vi "Timer2go.vi"() -> ()   [LabVIEW 2011]
uses:
  Control 1.ctl
panel:
  out "成功連結定時器":bool
  in  "stop 2":bool
  out "Today#2? \n(True=Enable)":bool
  out "now weekstring string":string
  out "after substring":string
  out "confilct ? (True=no conflict) 2":bool
  in  "Mon#2":bool
  in  "Tue#2":bool
  in  "Wed#2":bool
  in  "Thu#2":bool
  in  "Fri#2":bool
  in  "Sat#2":bool
  in  "Sun#2":bool
  in  "ON hour#2":i32
  in  "ON minute#2":i32
  in  "OFF hour#2":i32
  in  "OFF minute#2":i32
  out "week string#2":string
  out "ON hr+min#2":i32
  out "OFF hr+min#2":i32
  out "String":string
  out "path string":string
  out "read text":string
  out "CurrentPath":path=path "C:/Documents and Settings/TGI0362/My Documents/xUserData/LabVIEW_8.x/cmDVT_Factory-BBU-R5"
  in  "save":bool
  in  "error in":errorcluster
  in  "stop":bool
  out "error out 2":errorcluster
  out "VISA resource name out":refnum<visa-resource-name>
  out "error out":errorcluster
  out "VISA resource 2":refnum<visa-resource-name>
  out "定時器開啟":T1
  out "In Range?":bool
  out "hr+min":i32
  out "OFF hr+min#1":i32
  out "ON hr+min#1":i32
  out "Today#1? \n(True=Enable)":bool
  out "week string#1":string
  out "now week string":string
  out "confilct ? (True=no conflict)":bool
  in  "OFF minute#1":i32
  in  "OFF hour#1":i32
  in  "ON minute#1":i32
  in  "ON hour#1":i32
  in  "Sun#1":bool
  in  "Sat#1":bool
  in  "Fri#1":bool
  in  "Thu#1":bool
  in  "Wed#1":bool
  in  "Tue#1":bool
  in  "Mon#1":bool
  out "new picture":picture
  # "第一組\n\n\n第二組"
  # "："
  # "："
  # "："
  # "："
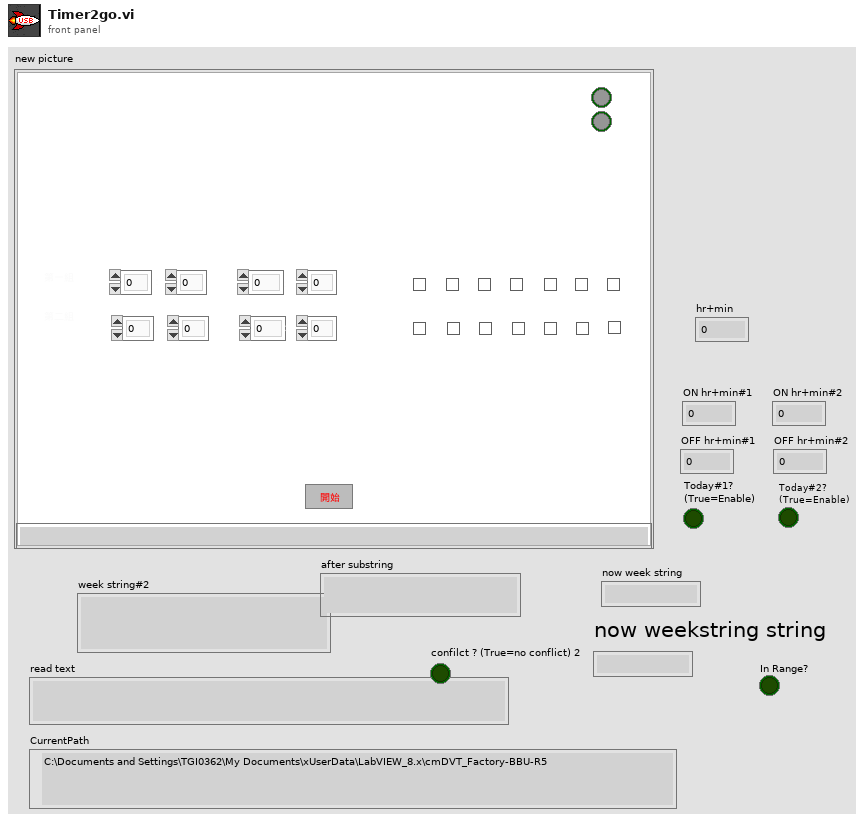
[diagram p1: front panel]
types:
  T1 = typedef "Control 1.ctl" = bool
  T2 = typedef "imagedata.ctl" = cluster{"image type":i32, "image depth":i32, "image":u8[], "mask":u8[], "colors":u32[], "Rectangle":cluster{"left":i16, "top":i16, "right":i16, "bottom":i16}}
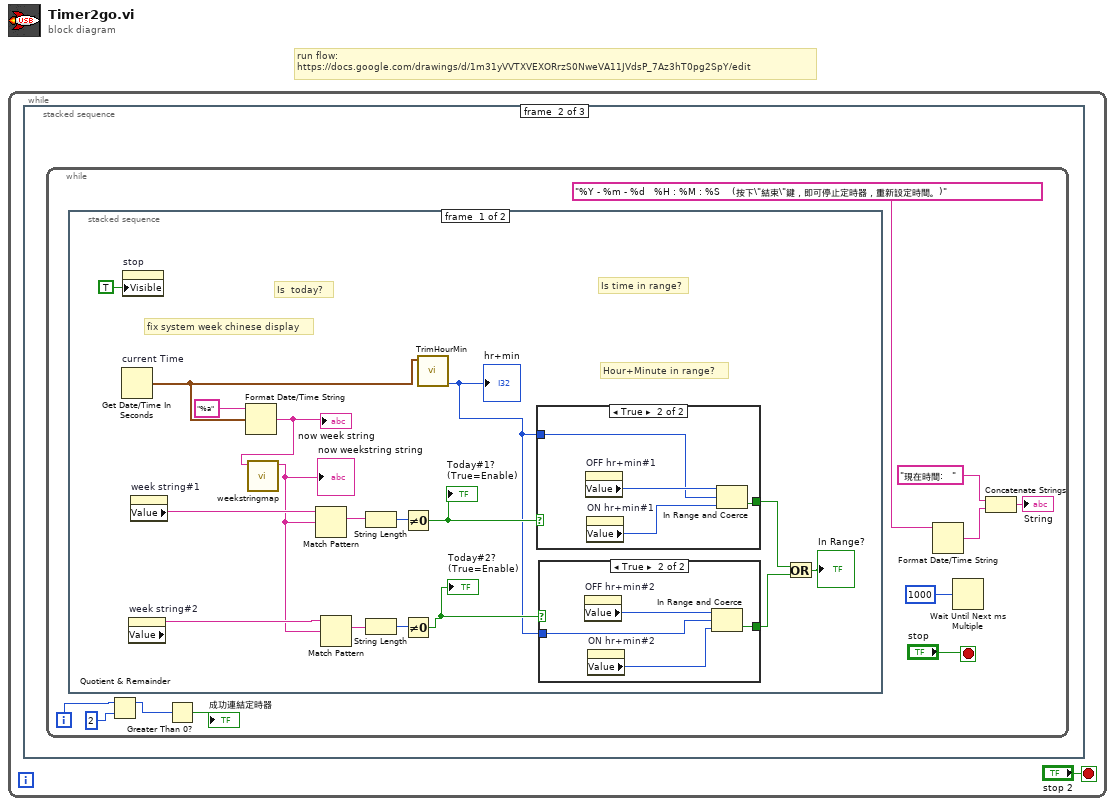
[diagram p0: block diagram]
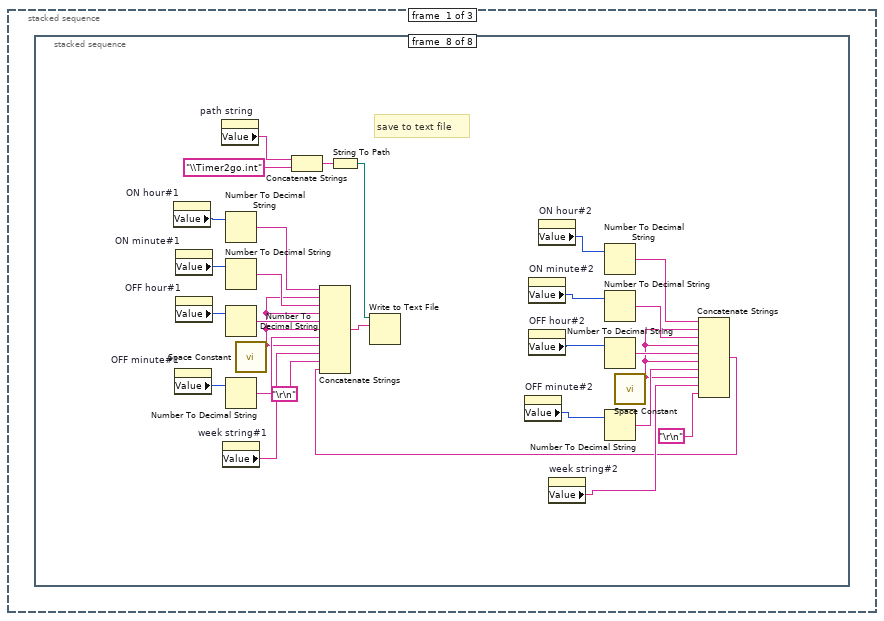
[diagram p2: hidden frame]
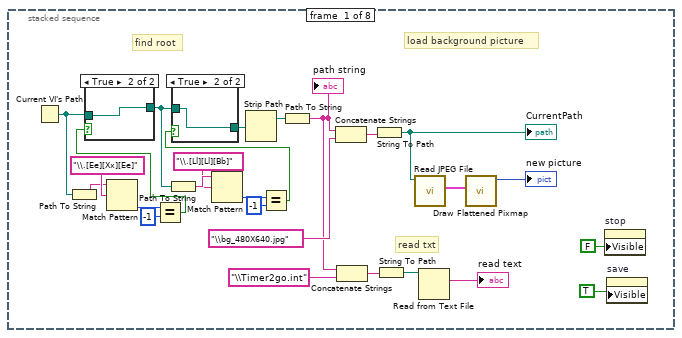
[diagram p3: hidden frame]
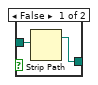
[diagram p4: hidden frame]
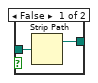
[diagram p5: hidden frame]
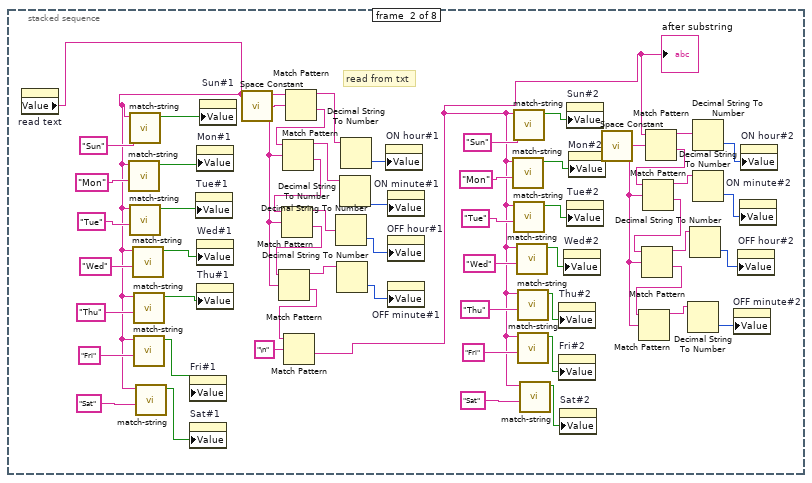
[diagram p6: hidden frame]
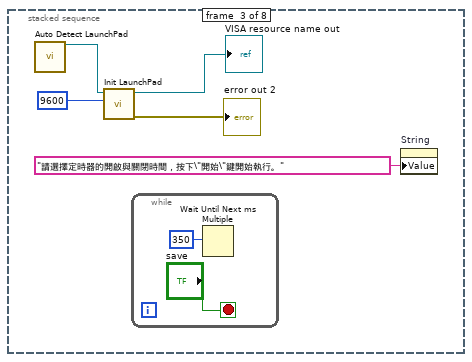
[diagram p7: hidden frame]
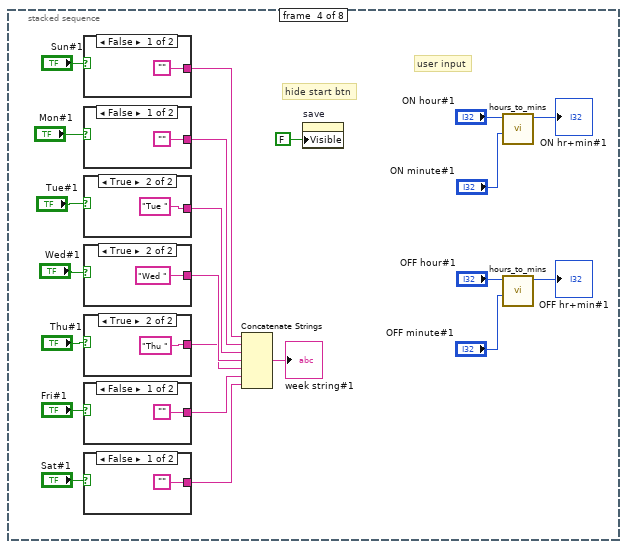
[diagram p8: hidden frame]
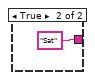
[diagram p9: hidden frame]
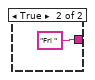
[diagram p10: hidden frame]
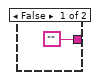
[diagram p11: hidden frame]
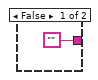
[diagram p12: hidden frame]
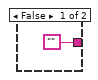
[diagram p13: hidden frame]
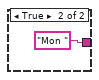
[diagram p14: hidden frame]
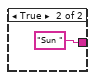
[diagram p15: hidden frame]
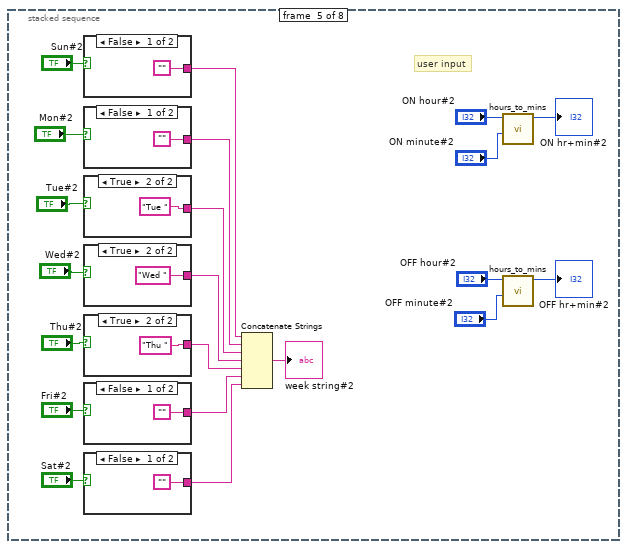
[diagram p16: hidden frame]
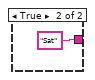
[diagram p17: hidden frame]
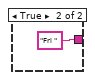
[diagram p18: hidden frame]
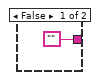
[diagram p19: hidden frame]
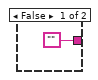
[diagram p20: hidden frame]
diagram:
  # "run flow:\nhttps://docs.google.com/drawings/d/1m31yVVTXVEXORrzS0NweVA11JVdsP_7Az3hT0pg2SpY/edit"
  n1 = while {
    stop <- "stop 2" stop-if-true
    n2 = stacked-sequence {
      frame #0 {
        n3 = stacked-sequence {
          frame #0 {
            # "read txt"
            # "load background picture"
            # "find root"
            n4 = Current VI's Path() -> (path=w16:path)
            n5 = Path To String(path=w16) -> (string=w15:string)
            n6 = Match Pattern(string=w15, regular expression="\\.[Ee][Xx][Ee]") -> (offset past match=w13:i32)  [unwired: 1 in, 3 out]
            n7 = Equal?(x=w13, y=-1) -> (x = y?=w25:bool)
            n8 = case shown="True" w25 {
              tunnel: [w31 w33] -> w22
              tunnel: w16 -> [w32 w33]
              frame False {
                n9 = Strip Path(path=w32) -> (stripped path=w31:path)  [unwired: 1 out]
              }
              frame True {
              }
            }
            n10 = Path To String(path=w22) -> (string=w19:string)
            n11 = Match Pattern(string=w19, regular expression="\\.[Ll][Ll][Bb]") -> (offset past match=w21:i32)  [unwired: 1 in, 3 out]
            n12 = Equal?(x=w21, y=-1) -> (x = y?=w24:bool)
            n13 = case shown="True" w24 {
              tunnel: [w28 w30] -> w23
              tunnel: w22 -> [w29 w30]
              frame False {
                n14 = Strip Path(path=w29) -> (stripped path=w28:path)  [unwired: 1 out]
              }
              frame True {
              }
            }
            n15 = Strip Path(path=w23) -> (stripped path=w12:path)  [unwired: 1 out]
            n16 = Path To String(path=w12) -> (string=w2:string)
            "path string" <- w2
            n17 = Concatenate Strings(w2, "\\bg_480X640.jpg") -> (w10:string)
            n18 = Concatenate Strings(w2, "\\Timer2go.int") -> (w5:string)
            n19 = String To Path(string=w10) -> (path=w9:path)
            "CurrentPath" <- w9
            n20 = String To Path(string=w5) -> (path=w4:path)
            n21 = call <vilib>:"Read JPEG File.vi"("path to JPEG file"=w9) -> ("image data"=w26:T2)  [unwired: 8 in, 2 out]
            n22 = Read from Text File(file (use dialog)=w4) -> (text=→"read text":string)  [unwired: 3 in, 3 out]
            n23 = call <vilib>:"Draw Flattened Pixmap.vi"("image data"=w26) -> ("new picture"=→"new picture":picture)  [unwired: 8 in]
            n24 = property on="stop" class="Bool"("Visible"=FALSE) -> ()  [unwired: 2 in, 2 out]
            n25 = property on="save" class="Bool"("Visible"=TRUE) -> ()  [unwired: 2 in, 2 out]
          }
          frame #1 {
            # "read from txt"
            n26 = property on="read text" class="Str"() -> ("Value"=w37:string)  [unwired: 2 in, 2 out]
            n27 = call "match-string.vi"("match string"="Mon", "String"=w37) -> ("match?(True=match)"=w76:bool)  [unwired: 9 in]
            n28 = call "match-string.vi"("match string"="Sun", "String"=w37) -> ("match?(True=match)"=w89:bool)  [unwired: 9 in]
            n29 = call "match-string.vi"("match string"="Tue", "String"=w37) -> ("match?(True=match)"=w77:bool)  [unwired: 9 in]
            n30 = call "match-string.vi"("match string"="Wed", "String"=w37) -> ("match?(True=match)"=w78:bool)  [unwired: 9 in]
            n31 = call "match-string.vi"("match string"="Thu", "String"=w37) -> ("match?(True=match)"=w79:bool)  [unwired: 9 in]
            n32 = call "match-string.vi"("match string"="Fri", "String"=w37) -> ("match?(True=match)"=w80:bool)  [unwired: 9 in]
            n33 = call "match-string.vi"("match string"="Sat", "String"=w37) -> ("match?(True=match)"=w81:bool)  [unwired: 9 in]
            n34 = property on="Fri#1" class="Bool (strict)"("Value"=w80) -> ()  [unwired: 2 in, 2 out]
            n35 = property on="Sat#1" class="Bool (strict)"("Value"=w81) -> ()  [unwired: 2 in, 2 out]
            n36 = property on="Tue#1" class="Bool (strict)"("Value"=w77) -> ()  [unwired: 2 in, 2 out]
            n37 = property on="Mon#1" class="Bool (strict)"("Value"=w76) -> ()  [unwired: 2 in, 2 out]
            n38 = property on="Wed#1" class="Bool (strict)"("Value"=w78) -> ()  [unwired: 2 in, 2 out]
            n39 = property on="Thu#1" class="Bool (strict)"("Value"=w79) -> ()  [unwired: 2 in, 2 out]
            n40 = property on="Sun#1" class="Bool (strict)"("Value"=w89) -> ()  [unwired: 2 in, 2 out]
            n41 = call <vilib>:"Space Constant.vi"() -> ("String"=w65:string)
            n42 = Match Pattern(string=w37, regular expression=w65) -> (before substring=w75:string, after substring=w73:string)  [unwired: 1 in, 2 out]
            n43 = Match Pattern(string=w73, regular expression=w65) -> (before substring=w72:string, after substring=w71:string)  [unwired: 1 in, 2 out]
            n44 = Match Pattern(string=w71, regular expression=w65) -> (before substring=w70:string, after substring=w67:string)  [unwired: 1 in, 2 out]
            n45 = Match Pattern(string=w67, regular expression=w65) -> (before substring=w66:string, after substring=w36:string)  [unwired: 1 in, 2 out]
            n46 = Match Pattern(string=w36, regular expression="\n") -> (after substring=w34:string)  [unwired: 1 in, 3 out]
            "after substring" <- w34
            n47 = Decimal String To Number(string=w70) -> (number=w69:i32)  [unwired: 2 in, 1 out]
            n48 = Decimal String To Number(string=w66) -> (number=w64:i32)  [unwired: 2 in, 1 out]
            n49 = Decimal String To Number(string=w72) -> (number=w68:i32)  [unwired: 2 in, 1 out]
            n50 = Decimal String To Number(string=w75) -> (number=w74:i32)  [unwired: 2 in, 1 out]
            n51 = property on="ON hour#1" class="DigNum (strict)"("Value"=w74) -> ()  [unwired: 2 in, 2 out]
            n52 = property on="ON minute#1" class="DigNum (strict)"("Value"=w68) -> ()  [unwired: 2 in, 2 out]
            n53 = property on="OFF hour#1" class="DigNum (strict)"("Value"=w69) -> ()  [unwired: 2 in, 2 out]
            n54 = property on="OFF minute#1" class="DigNum (strict)"("Value"=w64) -> ()  [unwired: 2 in, 2 out]
            n55 = call "match-string.vi"("match string"="Mon", "String"=w34) -> ("match?(True=match)"=w55:bool)  [unwired: 9 in]
            n56 = call "match-string.vi"("match string"="Sun", "String"=w34) -> ("match?(True=match)"=w56:bool)  [unwired: 9 in]
            n57 = call "match-string.vi"("match string"="Tue", "String"=w34) -> ("match?(True=match)"=w54:bool)  [unwired: 9 in]
            n58 = call "match-string.vi"("match string"="Wed", "String"=w34) -> ("match?(True=match)"=w53:bool)  [unwired: 9 in]
            n59 = call "match-string.vi"("match string"="Thu", "String"=w34) -> ("match?(True=match)"=w52:bool)  [unwired: 9 in]
            n60 = call "match-string.vi"("match string"="Fri", "String"=w34) -> ("match?(True=match)"=w51:bool)  [unwired: 9 in]
            n61 = call "match-string.vi"("match string"="Sat", "String"=w34) -> ("match?(True=match)"=w50:bool)  [unwired: 9 in]
            n62 = property on="Thu#2" class="Bool (strict)"("Value"=w52) -> ()  [unwired: 2 in, 2 out]
            n63 = property on="Fri#2" class="Bool (strict)"("Value"=w51) -> ()  [unwired: 2 in, 2 out]
            n64 = property on="Sat#2" class="Bool (strict)"("Value"=w50) -> ()  [unwired: 2 in, 2 out]
            n65 = property on="Wed#2" class="Bool (strict)"("Value"=w53) -> ()  [unwired: 2 in, 2 out]
            n66 = property on="Sun#2" class="Bool (strict)"("Value"=w56) -> ()  [unwired: 2 in, 2 out]
            n67 = property on="Tue#2" class="Bool (strict)"("Value"=w54) -> ()  [unwired: 2 in, 2 out]
            n68 = property on="Mon#2" class="Bool (strict)"("Value"=w55) -> ()  [unwired: 2 in, 2 out]
            n69 = call <vilib>:"Space Constant.vi"() -> ("String"=w38:string)
            n70 = Match Pattern(string=w34, regular expression=w38) -> (before substring=w49:string, after substring=w48:string)  [unwired: 1 in, 2 out]
            n71 = Match Pattern(string=w48, regular expression=w38) -> (before substring=w47:string, after substring=w46:string)  [unwired: 1 in, 2 out]
            n72 = Match Pattern(string=w46, regular expression=w38) -> (before substring=w45:string, after substring=w44:string)  [unwired: 1 in, 2 out]
            n73 = Match Pattern(string=w44, regular expression=w38) -> (before substring=w43:string)  [unwired: 1 in, 3 out]
            n74 = Decimal String To Number(string=w43) -> (number=w39:i32)  [unwired: 2 in, 1 out]
            n75 = Decimal String To Number(string=w45) -> (number=w40:i32)  [unwired: 2 in, 1 out]
            n76 = Decimal String To Number(string=w49) -> (number=w42:i32)  [unwired: 2 in, 1 out]
            n77 = Decimal String To Number(string=w47) -> (number=w41:i32)  [unwired: 2 in, 1 out]
            n78 = property on="OFF minute#2" class="DigNum (strict)"("Value"=w39) -> ()  [unwired: 2 in, 2 out]
            n79 = property on="OFF hour#2" class="DigNum (strict)"("Value"=w40) -> ()  [unwired: 2 in, 2 out]
            n80 = property on="ON minute#2" class="DigNum (strict)"("Value"=w41) -> ()  [unwired: 2 in, 2 out]
            n81 = property on="ON hour#2" class="DigNum (strict)"("Value"=w42) -> ()  [unwired: 2 in, 2 out]
          }
          frame #2 {
            n82 = call "Auto Detect LaunchPad.vi"() -> ("VISA resource"=w93:refnum<visa-resource-name>)  [unwired: 14 in, 1 out]
            n83 = call "Init LaunchPad.vi"("Baud Rate (9600)"=u32 9600, "VISA resource"=w93) -> ("error out"=→"error out 2":errorcluster, "VISA resource name out"=→"VISA resource name out":refnum<visa-resource-name>)  [unwired: 8 in]
            n84 = while {
              stop <- "save" stop-if-true
              n85 = Wait Until Next ms Multiple(millisecond multiple=u32 350) -> ()  [unwired: 1 out]
            }
            n86 = property on="String" class="Str"("Value"="請選擇定時器的開啟與關閉時間，按下\"開始\"鍵開始執行。" ("String")) -> ()  [unwired: 2 in, 2 out]
          }
          frame #3 {
            # "hide start btn"
            # "user input"
            n87 = case shown="False" "Sun#1" {
              tunnel: ["" "Sun "] -> w117
              frame False {
              }
              frame True {
              }
            }
            n88 = case shown="False" "Mon#1" {
              tunnel: ["" "Mon "] -> w110
              frame False {
              }
              frame True {
              }
            }
            n89 = case shown="True" "Tue#1" {
              tunnel: ["" "Tue "] -> w109
              frame False {
              }
              frame True {
              }
            }
            n90 = case shown="True" "Wed#1" {
              tunnel: ["" "Wed "] -> w108
              frame False {
              }
              frame True {
              }
            }
            n91 = case shown="True" "Thu#1" {
              tunnel: ["" "Thu "] -> w107
              frame False {
              }
              frame True {
              }
            }
            n92 = case shown="False" "Fri#1" {
              tunnel: ["" "Fri "] -> w106
              frame False {
              }
              frame True {
              }
            }
            n93 = case shown="False" "Sat#1" {
              tunnel: ["" "Sat"] -> w105
              frame False {
              }
              frame True {
              }
            }
            n94 = Concatenate Strings(w117, w110, w109, w108, w107, w106, w105) -> (→"week string#1":string)
            n95 = property on="save" class="Bool"("Visible"=FALSE) -> ()  [unwired: 2 in, 2 out]
            n96 = call "hours_to_mins.vi"("minute(00-59)"="ON minute#1", "hour(00-23)"="ON hour#1") -> ("hr+min"=→"ON hr+min#1":i32)  [unwired: 9 in]
            n97 = call "hours_to_mins.vi"("minute(00-59)"="OFF minute#1", "hour(00-23)"="OFF hour#1") -> ("hr+min"=→"OFF hr+min#1":i32)  [unwired: 9 in]
          }
          frame #4 {
            # "user input"
            n98 = case shown="False" "Sun#2" {
              tunnel: ["" "Sun "] -> w152
              frame False {
              }
              frame True {
              }
            }
            n99 = case shown="False" "Mon#2" {
              tunnel: ["" "Mon "] -> w145
              frame False {
              }
              frame True {
              }
            }
            n100 = case shown="True" "Tue#2" {
              tunnel: ["" "Tue "] -> w144
              frame False {
              }
              frame True {
              }
            }
            n101 = case shown="True" "Wed#2" {
              tunnel: ["" "Wed "] -> w143
              frame False {
              }
              frame True {
              }
            }
            n102 = case shown="True" "Thu#2" {
              tunnel: ["" "Thu "] -> w142
              frame False {
              }
              frame True {
              }
            }
            n103 = case shown="False" "Fri#2" {
              tunnel: ["" "Fri "] -> w141
              frame False {
              }
              frame True {
              }
            }
            n104 = case shown="False" "Sat#2" {
              tunnel: ["" "Sat"] -> w140
              frame False {
              }
              frame True {
              }
            }
            n105 = Concatenate Strings(w152, w145, w144, w143, w142, w141, w140) -> (→"week string#2":string)
            n106 = call "hours_to_mins.vi"("minute(00-59)"="ON minute#2", "hour(00-23)"="ON hour#2") -> ("hr+min"=→"ON hr+min#2":i32)  [unwired: 9 in]
            n107 = call "hours_to_mins.vi"("minute(00-59)"="OFF minute#2", "hour(00-23)"="OFF hour#2") -> ("hr+min"=→"OFF hr+min#2":i32)  [unwired: 9 in]
          }
          frame #5 {
            # "check Set Time conflict"
            n108 = property on="ON hour#1" class="DigNum (strict)"() -> ("Value"=w187:i32)  [unwired: 2 in, 2 out]
            n109 = property on="OFF hour#1" class="DigNum (strict)"() -> ("Value"=w190:i32)  [unwired: 2 in, 2 out]
            n110 = property on="ON minute#1" class="DigNum (strict)"() -> ("Value"=w184:i32)  [unwired: 2 in, 2 out]
            n111 = property on="OFF minute#1" class="DigNum (strict)"() -> ("Value"=w181:i32)  [unwired: 2 in, 2 out]
            n112 = Equal?(x=w190, y=0) -> (x = y?=w192:bool)
            n113 = Equal?(x=w187, y=0) -> (x = y?=w189:bool)
            n114 = case shown="False" w192 {
              tunnel: [w203 24] -> w177
              tunnel: w190 -> [w203 _]
              frame False {
              }
              frame True {
              }
            }
            n115 = case shown="False" w189 {
              tunnel: [w201 24] -> w171
              tunnel: w187 -> [w201 _]
              frame False {
              }
              frame True {
              }
            }
            n116 = Equal?(x=w181, y=0) -> (x = y?=w183:bool)
            n117 = Equal?(x=w184, y=0) -> (x = y?=w186:bool)
            n118 = case shown="False" w183 {
              tunnel: [w197 60] -> w174
              tunnel: w181 -> [w197 _]
              frame False {
              }
              frame True {
              }
            }
            n119 = case shown="False" w186 {
              tunnel: [w199 60] -> w169
              tunnel: w184 -> [w199 _]
              frame False {
              }
              frame True {
              }
            }
            n120 = Multiply(x=w177, y=60) -> (x*y=w175:i32)
            n121 = Multiply(x=w171, y=60) -> (x*y=w170:i32)
            n122 = Add(x=w175, y=w174) -> (x+y=w173:i32)
            n123 = Add(x=w170, y=w169) -> (x+y=w168:i32)
            n124 = Subtract(x=w177, y=w171) -> (x-y=w194:i32)
            n125 = Subtract(x=w173, y=w168) -> (x-y=w193:i32)
            n126 = Greater Or Equal To 0?(x=w194) -> (x >= 0?=w180:bool)
            n127 = Greater Than 0?(x=w193) -> (x > 0?=w179:bool)
            n128 = And(x=w180, y=w179) -> (x .and. y?=w178:bool)
            "confilct ? (True=no conflict)" <- w178
            n129 = case shown="True" w178 {
              frame False {
                n130 = One Button Dialog(message="time confilct!!") -> (true=w195:bool)  [unwired: 1 in]
                n131 = Stop(stop? (T)=w195) -> ()
              }
              frame True {
              }
            }
          }
          frame #6 {
            # "check Set Time conflict"
            n132 = property on="OFF minute#2" class="DigNum (strict)"() -> ("Value"=w207:i32)  [unwired: 2 in, 2 out]
            n133 = property on="ON hour#2" class="DigNum (strict)"() -> ("Value"=w206:i32)  [unwired: 2 in, 2 out]
            n134 = property on="OFF hour#2" class="DigNum (strict)"() -> ("Value"=w208:i32)  [unwired: 2 in, 2 out]
            n135 = property on="ON minute#2" class="DigNum (strict)"() -> ("Value"=w205:i32)  [unwired: 2 in, 2 out]
            n136 = Equal?(x=w208, y=0) -> (x = y?=w229:bool)
            n137 = Equal?(x=w206, y=0) -> (x = y?=w227:bool)
            n138 = case shown="False" w229 {
              tunnel: [w240 24] -> w218
              tunnel: w208 -> [w240 _]
              frame False {
              }
              frame True {
              }
            }
            n139 = case shown="False" w227 {
              tunnel: [w238 24] -> w212
              tunnel: w206 -> [w238 _]
              frame False {
              }
              frame True {
              }
            }
            n140 = Equal?(x=w207, y=0) -> (x = y?=w223:bool)
            n141 = Equal?(x=w205, y=0) -> (x = y?=w225:bool)
            n142 = case shown="False" w223 {
              tunnel: [w234 60] -> w215
              tunnel: w207 -> [w234 _]
              frame False {
              }
              frame True {
              }
            }
            n143 = case shown="False" w225 {
              tunnel: [w236 60] -> w210
              tunnel: w205 -> [w236 _]
              frame False {
              }
              frame True {
              }
            }
            n144 = Multiply(x=w218, y=60) -> (x*y=w216:i32)
            n145 = Multiply(x=w212, y=60) -> (x*y=w211:i32)
            n146 = Add(x=w216, y=w215) -> (x+y=w214:i32)
            n147 = Add(x=w211, y=w210) -> (x+y=w209:i32)
            n148 = Subtract(x=w218, y=w212) -> (x-y=w231:i32)
            n149 = Subtract(x=w214, y=w209) -> (x-y=w230:i32)
            n150 = Greater Or Equal To 0?(x=w231) -> (x >= 0?=w221:bool)
            n151 = Greater Than 0?(x=w230) -> (x > 0?=w220:bool)
            n152 = And(x=w221, y=w220) -> (x .and. y?=w219:bool)
            "confilct ? (True=no conflict) 2" <- w219
            n153 = case shown="True" w219 {
              frame False {
                n154 = One Button Dialog(message="time confilct!!") -> (true=w232:bool)  [unwired: 1 in]
                n155 = Stop(stop? (T)=w232) -> ()
              }
              frame True {
              }
            }
          }
          frame #7 {
            # "save to text file"
            n156 = property on="ON hour#1" class="DigNum (strict)"() -> ("Value"=w258:i32)  [unwired: 2 in, 2 out]
            n157 = property on="OFF minute#1" class="DigNum (strict)"() -> ("Value"=w255:i32)  [unwired: 2 in, 2 out]
            n158 = property on="ON minute#1" class="DigNum (strict)"() -> ("Value"=w257:i32)  [unwired: 2 in, 2 out]
            n159 = property on="OFF hour#1" class="DigNum (strict)"() -> ("Value"=w256:i32)  [unwired: 2 in, 2 out]
            n160 = property on="path string" class="Str"() -> ("Value"=w260:string)  [unwired: 2 in, 2 out]
            n161 = property on="week string#1" class="Str"() -> ("Value"=w265:string)  [unwired: 2 in, 2 out]
            n162 = Number To Decimal String(number=w258) -> (decimal integer string=w269:string)  [unwired: 1 in]
            n163 = Number To Decimal String(number=w257) -> (decimal integer string=w268:string)  [unwired: 1 in]
            n164 = Number To Decimal String(number=w256) -> (decimal integer string=w267:string)  [unwired: 1 in]
            n165 = Number To Decimal String(number=w255) -> (decimal integer string=w266:string)  [unwired: 1 in]
            n166 = call <vilib>:"Space Constant.vi"() -> ("String"=w264:string)
            n167 = Concatenate Strings(w260, "\\Timer2go.int") -> (w261:string)
            n168 = String To Path(string=w261) -> (path=w259:path)
            n169 = property on="OFF minute#2" class="DigNum (strict)"() -> ("Value"=w246:i32)  [unwired: 2 in, 2 out]
            n170 = property on="ON minute#2" class="DigNum (strict)"() -> ("Value"=w248:i32)  [unwired: 2 in, 2 out]
            n171 = property on="OFF hour#2" class="DigNum (strict)"() -> ("Value"=w247:i32)  [unwired: 2 in, 2 out]
            n172 = property on="ON hour#2" class="DigNum (strict)"() -> ("Value"=w249:i32)  [unwired: 2 in, 2 out]
            n173 = property on="week string#2" class="Str"() -> ("Value"=w245:string)  [unwired: 2 in, 2 out]
            n174 = Number To Decimal String(number=w249) -> (decimal integer string=w254:string)  [unwired: 1 in]
            n175 = Number To Decimal String(number=w248) -> (decimal integer string=w253:string)  [unwired: 1 in]
            n176 = Number To Decimal String(number=w247) -> (decimal integer string=w252:string)  [unwired: 1 in]
            n177 = Number To Decimal String(number=w246) -> (decimal integer string=w251:string)  [unwired: 1 in]
            n178 = call <vilib>:"Space Constant.vi"() -> ("String"=w250:string)
            n179 = Concatenate Strings(w254, w250, w253, w250, w252, w250, w251, w250, w245, "\r\n") -> (w244:string)
            n180 = Concatenate Strings(w269, w264, w268, w264, w267, w264, w266, w264, w265, "\r\n", w244) -> (w263:string)
            n181 = Write to Text File(file (use dialog)=w259, text=w263) -> ()  [unwired: 2 in, 3 out]
          }
        }
      }
      frame #1 {
        n182 = while {
          i -> [w273]
          stop <- "stop" stop-if-true
          n183 = stacked-sequence {
            frame #0 {
              # "Hour+Minute in range?"
              # "fix system week chinese display"
              # "Is time in range?"
              # "Is  today?"
              n184 = Get Date/Time In Seconds "current Time"() -> (seconds since 1Jan1904=w290:timestamp)
              n185 = property on="stop" class="Bool"("Visible"=TRUE) -> ()  [unwired: 2 in, 2 out]
              n186 = property on="week string#2" class="Str"() -> ("Value"=w289:string)  [unwired: 2 in, 2 out]
              n187 = property on="week string#1" class="Str"() -> ("Value"=w295:string)  [unwired: 2 in, 2 out]
              n188 = Format Date/Time String(time format string (%c)="%a", seconds (now)=w290) -> (date/time string=w280:string)  [unwired: 1 in]
              "now week string" <- w280
              n189 = call "weekstringmap.vi"("now weekstring input"=w280) -> ("now weekstring string"=w281:string)  [unwired: 10 in]
              "now weekstring string" <- w281
              n190 = Match Pattern(string=w295, regular expression=w281) -> (match substring=w294:string)  [unwired: 1 in, 3 out]
              n191 = Match Pattern(string=w289, regular expression=w281) -> (match substring=w287:string)  [unwired: 1 in, 3 out]
              n192 = String Length(string=w294) -> (length=w293:i32)
              n193 = String Length(string=w287) -> (length=w288:i32)
              n194 = Not Equal To 0?(x=w293) -> (x != 0?=w291:bool)
              "Today#1? \n(True=Enable)" <- w291
              n195 = Not Equal To 0?(x=w288) -> (x != 0?=w285:bool)
              "Today#2? \n(True=Enable)" <- w285
              n196 = call "TrimHourMin.vi"("Time"=w290) -> ("hr+min"=w284:i32)  [unwired: 8 in, 2 out]
              "hr+min" <- w284
              n197 = case shown="True" w291 {
                selector: w291 -> [w302 _]
                tunnel: [w302 w303] -> w286
                tunnel: w284 -> [_ w304]
                frame False {
                }
                frame True {
                  n198 = property on="OFF hr+min#1" class="DigNum (strict)"() -> ("Value"=w305:i32)  [unwired: 2 in, 2 out]
                  n199 = property on="ON hr+min#1" class="DigNum (strict)"() -> ("Value"=w306:i32)  [unwired: 2 in, 2 out]
                  n200 = In Range and Coerce(upper limit=w305, x=w304, lower limit=w306) -> (In Range?=w303:bool)  [unwired: 1 out]
                }
              }
              n201 = case shown="True" w285 {
                selector: w285 -> [w297 _]
                tunnel: w284 -> [_ w299]
                tunnel: [w297 w298] -> w283
                frame False {
                }
                frame True {
                  n202 = property on="OFF hr+min#2" class="DigNum (strict)"() -> ("Value"=w300:i32)  [unwired: 2 in, 2 out]
                  n203 = property on="ON hr+min#2" class="DigNum (strict)"() -> ("Value"=w301:i32)  [unwired: 2 in, 2 out]
                  n204 = In Range and Coerce(upper limit=w300, x=w299, lower limit=w301) -> (In Range?=w298:bool)  [unwired: 1 out]
                }
              }
              n205 = Or(x=w286, y=w283) -> (x .or. y?=→"In Range?":bool)
            }
            frame #1 {
              # "LabVIEW Interface for LaunchPad (LILP_MSP430G2553) v1\n#define            M_D0        0x30   // Char ASCII \"0\"\n#define            M_A4        0x34   // Char ASCII \"4\""
              # "1000"
              # "check P1.0 status by P1.4 analog (if ON P1.4=1000, if OFF=0000)"
              n206 = property on="VISA resource name out" class="VISAName"() -> ("Value"=w309:refnum<visa-resource-name>)  [unwired: 2 in, 2 out]
              n207 = property on="error out 2" class="Clust (strict)"() -> ("Value"=w308:errorcluster)  [unwired: 2 in, 2 out]
              n208 = call "Send Receive LaunchPad.vi"("VISA resource"=w309, "write buffer"="4", "Bytes To Read (0)"=u8 2, "Max Retries  (10)"=1, "error in"=w308) -> ("VISA resource 2"=→"VISA resource 2":refnum<visa-resource-name>, "Read Buffer"=w315:string, "error out"=→"error out":errorcluster)  [unwired: 8 in]
              n209 = call "ADC10 LaunchPad.vi"("string"=w315) -> ("ADCvalue"=w313:u16)  [unwired: 9 in, 1 out]
              n210 = Greater?(x=w313, y=u16 900) -> (0:w307:bool)
              "定時器開啟" <- w307
              n211 = case shown="True" w307 {
                frame False {
                  n212 = property on="In Range?" class="Bool (strict)"() -> ("Value"=w318:bool)  [unwired: 2 in, 2 out]
                  n213 = case shown="True" w318 {
                    frame False {
                      # "do nothing"
                    }
                    frame True {
                      # "need toggle to turn ON"
                      n214 = property on="VISA resource 2" class="VISAName"() -> ("Value"=w321:refnum<visa-resource-name>)  [unwired: 2 in, 2 out]
                      n215 = property on="error out" class="Clust (strict)"() -> ("Value"=w320:errorcluster)  [unwired: 2 in, 2 out]
                      n216 = call "Send Receive LaunchPad.vi"("VISA resource"=w321, "write buffer"="0", "Bytes To Read (0)"=u8 2, "Max Retries  (10)"=1, "error in"=w320) -> ("error out"=w319:errorcluster)  [unwired: 8 in, 2 out]
                      n217 = property on="error in" class="Clust (strict)"("Value"=w319) -> ()  [unwired: 2 in, 2 out]
                    }
                  }
                }
                frame True {
                  n218 = property on="In Range?" class="Bool (strict)"() -> ("Value"=w325:bool)  [unwired: 2 in, 2 out]
                  n219 = case shown="False" w325 {
                    frame False {
                      # "in error action , try to toggle trun off"
                      n220 = property on="VISA resource 2" class="VISAName"() -> ("Value"=w328:refnum<visa-resource-name>)  [unwired: 2 in, 2 out]
                      n221 = property on="error out" class="Clust (strict)"() -> ("Value"=w327:errorcluster)  [unwired: 2 in, 2 out]
                      n222 = call "Send Receive LaunchPad.vi"("VISA resource"=w328, "write buffer"="0", "Bytes To Read (0)"=u8 2, "Max Retries  (10)"=1, "error in"=w327) -> ("error out"=w326:errorcluster)  [unwired: 8 in, 2 out]
                      n223 = property on="error in" class="Clust (strict)"("Value"=w326) -> ()  [unwired: 2 in, 2 out]
                    }
                    frame True {
                      # "do nothing"
                    }
                  }
                }
              }
            }
          }
          n224 = Quotient & Remainder(x=w273, y=2) -> (x-y*floor(x/y)=w271:i32)  [unwired: 1 out]
          n225 = Greater Than 0?(x=w271) -> (x > 0?=→"成功連結定時器":bool)
          n226 = Format Date/Time String(time format string (%c)="%Y - %m - %d   %H : %M : %S 　(按下\"結束\"鍵，即可停止定時器，重新設定時間。)") -> (date/time string=w276:string)  [unwired: 2 in]
          n227 = Wait Until Next ms Multiple(millisecond multiple=u32 1000) -> ()  [unwired: 1 out]
          n228 = Concatenate Strings("現在時間:   ", w276) -> (→"String":string)
        }
      }
      frame #2 {
        # "exit LP"
        # "show tools bar status"
        # "save to text file"
        n229 = property on="VISA resource name out" class="VISAName"() -> ("Value"=w361:refnum<visa-resource-name>)  [unwired: 2 in, 2 out]
        n230 = call "Close LaunchPad.vi"("VISA resource name"=w361, "error in"="error in") -> ()  [unwired: 13 in, 1 out]
        n231 = property on="ON hour#1" class="DigNum (strict)"() -> ("Value"=w348:i32)  [unwired: 2 in, 2 out]
        n232 = property on="OFF minute#1" class="DigNum (strict)"() -> ("Value"=w345:i32)  [unwired: 2 in, 2 out]
        n233 = property on="ON minute#1" class="DigNum (strict)"() -> ("Value"=w347:i32)  [unwired: 2 in, 2 out]
        n234 = property on="OFF hour#1" class="DigNum (strict)"() -> ("Value"=w346:i32)  [unwired: 2 in, 2 out]
        n235 = property on="path string" class="Str"() -> ("Value"=w350:string)  [unwired: 2 in, 2 out]
        n236 = property on="week string#1" class="Str"() -> ("Value"=w355:string)  [unwired: 2 in, 2 out]
        n237 = Number To Decimal String(number=w348) -> (decimal integer string=w359:string)  [unwired: 1 in]
        n238 = Number To Decimal String(number=w347) -> (decimal integer string=w358:string)  [unwired: 1 in]
        n239 = Number To Decimal String(number=w346) -> (decimal integer string=w357:string)  [unwired: 1 in]
        n240 = Number To Decimal String(number=w345) -> (decimal integer string=w356:string)  [unwired: 1 in]
        n241 = call <vilib>:"Space Constant.vi"() -> ("String"=w354:string)
        n242 = Concatenate Strings(w350, "\\Timer2go.int") -> (w351:string)
        n243 = String To Path(string=w351) -> (path=w349:path)
        n244 = property on="Save/Start" class="Bool"("Visible"=TRUE) -> ()  [unwired: 2 in, 2 out]
        n245 = property on="OFF minute#2" class="DigNum (strict)"() -> ("Value"=w336:i32)  [unwired: 2 in, 2 out]
        n246 = property on="ON minute#2" class="DigNum (strict)"() -> ("Value"=w338:i32)  [unwired: 2 in, 2 out]
        n247 = property on="OFF hour#2" class="DigNum (strict)"() -> ("Value"=w337:i32)  [unwired: 2 in, 2 out]
        n248 = property on="ON hour#2" class="DigNum (strict)"() -> ("Value"=w339:i32)  [unwired: 2 in, 2 out]
        n249 = property on="week string#2" class="Str"() -> ("Value"=w335:string)  [unwired: 2 in, 2 out]
        n250 = Number To Decimal String(number=w339) -> (decimal integer string=w344:string)  [unwired: 1 in]
        n251 = Number To Decimal String(number=w338) -> (decimal integer string=w343:string)  [unwired: 1 in]
        n252 = Number To Decimal String(number=w337) -> (decimal integer string=w342:string)  [unwired: 1 in]
        n253 = Number To Decimal String(number=w336) -> (decimal integer string=w341:string)  [unwired: 1 in]
        n254 = call <vilib>:"Space Constant.vi"() -> ("String"=w340:string)
        n255 = Concatenate Strings(w344, w340, w343, w340, w342, w340, w341, w340, w335, "\r\n") -> (w334:string)
        n256 = Concatenate Strings(w359, w354, w358, w354, w357, w354, w356, w354, w355, "\r\n", w334) -> (w353:string)
        n257 = Write to Text File(file (use dialog)=w349, text=w353) -> ()  [unwired: 2 in, 3 out]
      }
    }
  }
